vi "WoF_PID.vi"(5 "SimMode":bool, 6 "Reset":bool, 7 "Desired":dbl, 8 "D":dbl, 9 "I":dbl, 10 "P":dbl min=0.0 step=0.05, 11 "Actual":dbl) -> (3 "Control Effort":dbl)   [LabVIEW 2013]
panel:
  out "D Control":dbl(knob) scale=-1.5..1.5
  out "I Control":dbl
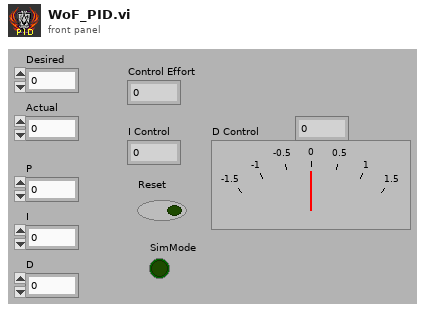
[diagram p1: front panel]
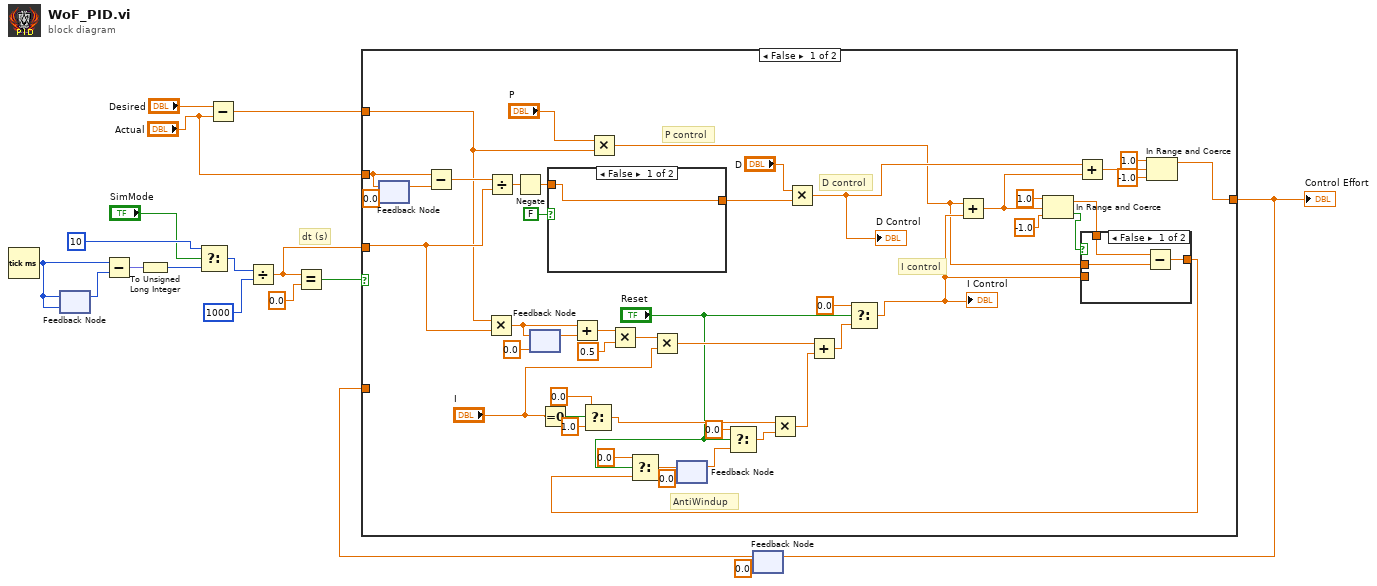
[diagram p0: block diagram]
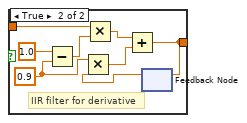
[diagram p2: hidden frame]
diagram:
  # "dt (s)"
  n1 = Tick Count (ms)() -> (millisecond timer value=w4:u32)
  n2 = feedback-in #1(w4) -> ()
  n3 = feedback #1(w4) -> (w5:u32)
  n4 = Subtract(x=w4, y=w5) -> (x-y=w3:fxp<+/-,32,32>)
  n5 = To Unsigned Long Integer(number=w3) -> (unsigned 32bit integer=w2:u32)
  n6 = Select(t=u32 10 ("x"), s="SimMode", f=w2) -> (s? t:f=w7:u32)
  n7 = Subtract(x="Desired", y="Actual") -> (x-y=w15:dbl)
  n8 = Divide(x=w7, y=u32 1000) -> (x/y=w11:dbl)
  n9 = Equal?(x=w11, y=0.0) -> (x = y?=w10:bool)
  n10 = feedback #2(0.0 ("upper limit")) -> (w13:dbl)
  n11 = case shown="False" w10 {
    tunnel: w15 -> [w56 _]
    tunnel: w11 -> [w58 _]
    tunnel: [w44 w78] -> w14
    tunnel: w13 -> [_ w78]
    tunnel: "Actual" -> [w55 _]
    frame False {
      # "AntiWindup"
      # "I control"
      # "D control"
      # "P control"
      n12 = feedback-in #3(w55) -> ()
      n13 = feedback #3(0.0 ("Actual")) -> (w60:dbl)
      n14 = Subtract(x=w55, y=w60) -> (x-y=w61:dbl)
      n15 = Multiply(x=w56, y=w58) -> (x*y=w40:dbl)
      n16 = Divide(x=w61, y=w58) -> (x/y=w53:dbl)
      n17 = Negate(x=w53) -> (-x=w51:dbl)
      n18 = feedback #4(0.0) -> (w39:dbl)
      n19 = feedback-in #4(w40) -> ()
      n20 = Equal To 0?(x="I") -> (x = 0?=w28:bool)
      n21 = case shown="False" FALSE {
        tunnel: [w65 w68] -> w52
        tunnel: w51 -> [w65 w67]
        frame False {
        }
        frame True {
          w69 = 0.9 ("y")
          # "IIR filter for derivative"
          n22 = Subtract(x=1.0, y=w69) -> (x-y=w66:dbl)
          n23 = Multiply(x=w67, y=w66) -> (x*y=w73:dbl)
          n24 = feedback #5() -> (w71:dbl)  [unwired: 1 out]
          n25 = Multiply(x=w69, y=w71) -> (x*y=w72:dbl)
          n26 = Add(x=w73, y=w72) -> (x+y=w68:dbl)
          n27 = feedback-in #5(w68) -> ()
        }
      }
      n28 = Add(x=w40, y=w39) -> (x+y=w38:dbl)
      n29 = Select(t=0.0, s=w28, f=1.0) -> (s? t:f=w25:dbl)
      n30 = Multiply(x="P", y=w56) -> (x*y=w31:dbl)
      n31 = Multiply(x=w38, y=0.5) -> (x*y=w35:dbl)
      n32 = Multiply(x=w35, y="I") -> (x*y=w34:dbl)
      n33 = feedback #6(0.0) -> (w19:dbl)
      n34 = Select(t=0.0, s="Reset", f=w19) -> (s? t:f=w24:dbl)
      n35 = Multiply(x=w25, y=w24) -> (x*y=w30:dbl)
      n36 = Multiply(x="D", y=w52) -> (x*y=w48:dbl)
      "D Control" <- w48
      n37 = Add(x=w34, y=w30) -> (x+y=w33:dbl)
      n38 = Select(t=0.0, s="Reset", f=w33) -> (s? t:f=w32:dbl)
      "I Control" <- w32
      n39 = Add(x=w31, y=w32) -> (x+y=w41:dbl)
      n40 = In Range and Coerce(upper limit=1.0, x=w41, lower limit=-1.0) -> (coerced(x)=w49:dbl, In Range?=w50:bool)
      n41 = Add(x=w48, y=w41) -> (x+y=w47:dbl)
      n42 = case shown="False" w50 {
        tunnel: [w76 w77] -> w20
        tunnel: w49 -> [w75 _]
        tunnel: w31 -> [w74 _]
        tunnel: w32 -> [_ w77]
        frame False {
          n43 = Subtract(x=w75, y=w74) -> (x-y=w76:dbl)
        }
        frame True {
        }
      }
      n44 = Select(t=0.0, s="Reset", f=w20) -> (s? t:f=w22:dbl)
      n45 = feedback-in #6(w22) -> ()
      n46 = In Range and Coerce(upper limit=1.0, x=w47, lower limit=-1.0) -> (coerced(x)=w44:dbl)  [unwired: 1 out]
    }
    frame True {
    }
  }
  "Control Effort" <- w14
  n47 = feedback-in #2(w14) -> ()
